vi "BRig_dataMTrig_Laser_c_l1.vi"() -> (2 "output_Laser_c_l1":i32)   [LabVIEW 2014]
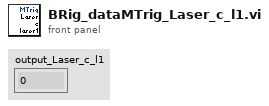
[diagram p1: front panel]
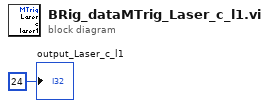
[diagram p0: block diagram]
diagram:
  "output_Laser_c_l1" <- 24 ("output_iBlock")
